vi "Disable All Buttons(Motor Movement).vi"(8 "error in (no error)":errorcluster, 11 "ZenGage v3.0 UI in":refnum<class "ZenGage v3.0 UI.lvclass">) -> (0 "error out":errorcluster, 3 "ZenGage v3.0 UI out":refnum<class "ZenGage v3.0 UI.lvclass">)   [LabVIEW 2015, in "ZenGage v3.0 UI.lvclass"]
uses:
  ZenGage v3.0 UI.lvclass
  ZenGage v3.0 UI.lvclass/ZenGage v3.0 UI.ctl
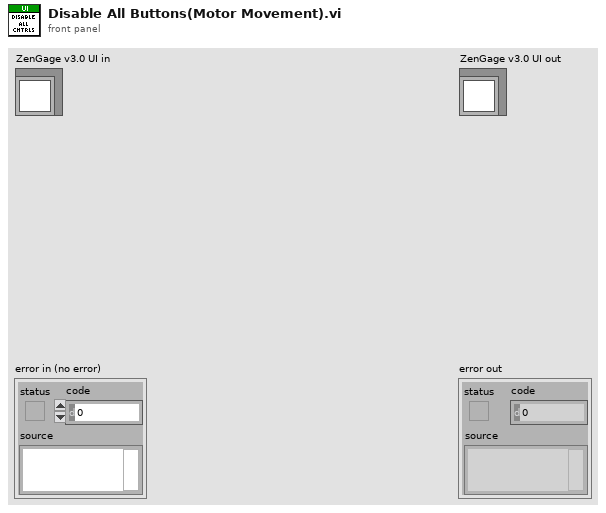
[diagram p1: front panel]
types:
  T1 = enum32{"Analytics", "Blank", "Diagnostics", "Run", "Edit Tolerance Settings"}
  T2 = enum8{"Enabled", "Disabled", "Disabled and Grayed Out"}
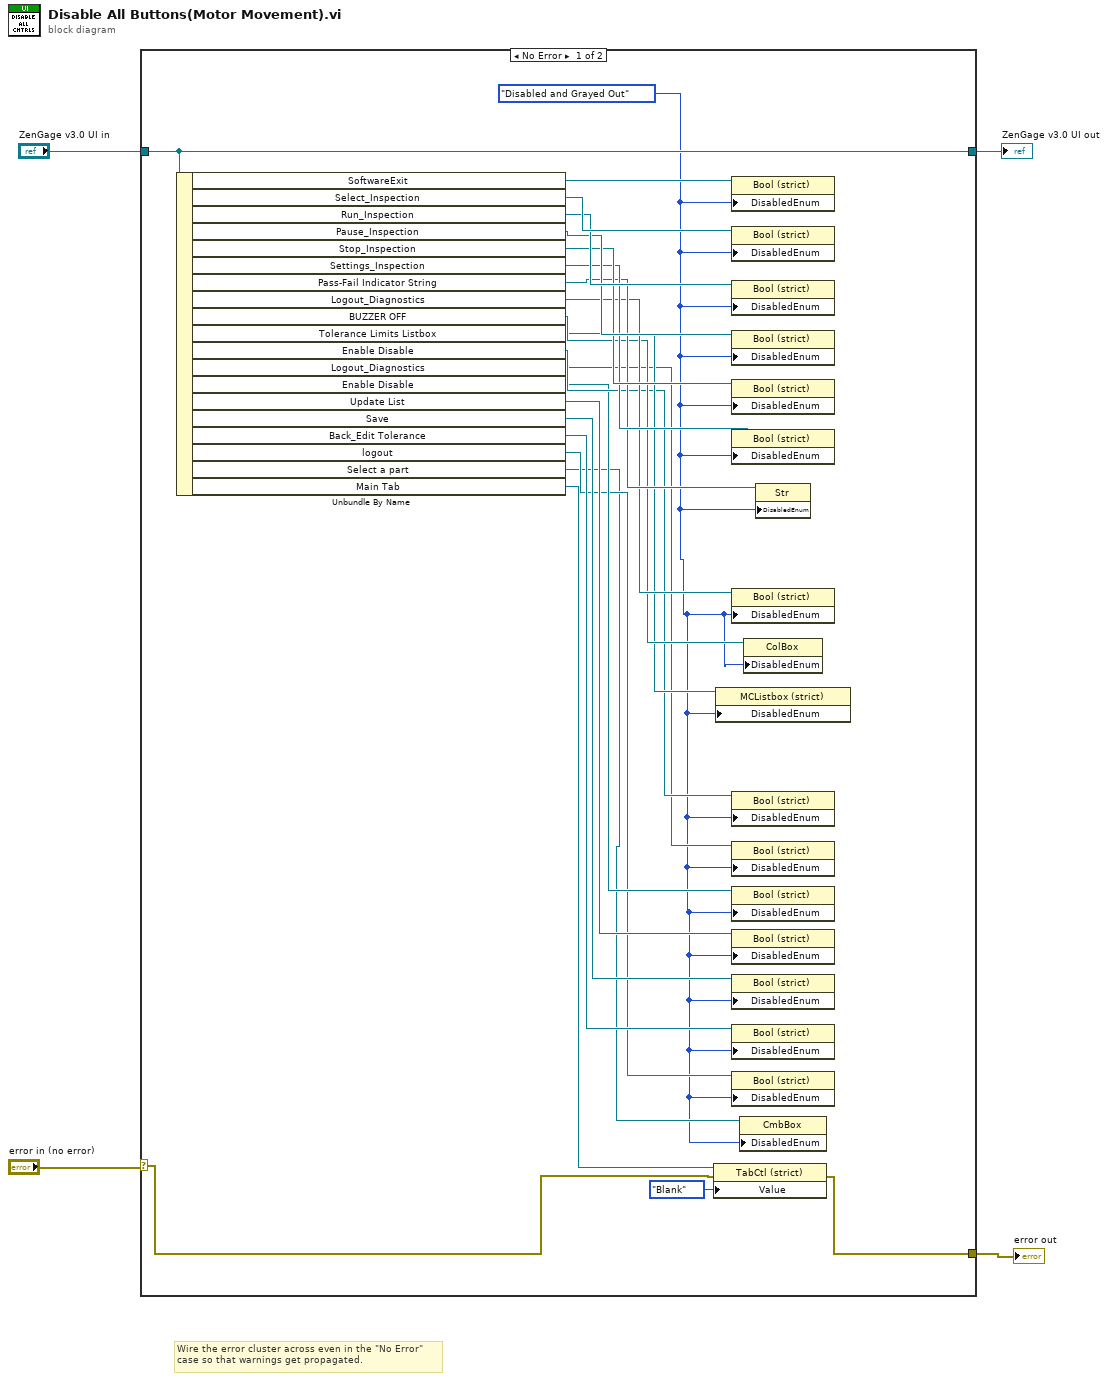
[diagram p0: block diagram]
diagram:
  # "Wire the error cluster across even in the \"No Error\"\ncase so that warnings get propagated."
  n1 = case shown="No Error" "error in (no error)" {
    selector: "error in (no error)" -> [w8 w30]
    tunnel: [w7 w30] -> w3
    tunnel: [w28 w29] -> w1
    tunnel: "ZenGage v3.0 UI in" -> [w28 w29]
    frame No Error {
      w5 = T2."Disabled and Grayed Out" ("Disabled")
      n2 = Unbundle By Name(w28) -> ("SoftwareExit"=w27:refnum<vi>, "Select_Inspection"=w26:refnum<vi>, "Run_Inspection"=w25:refnum<vi>, "Pause_Inspection"=w24:refnum<vi>, "Stop_Inspection"=w23:refnum<vi>, "Settings_Inspection"=w22:refnum<vi>, "Pass-Fail Indicator String"=w21:refnum<vi>, "Logout_Diagnostics"=w20:refnum<vi>, "BUZZER OFF"=w19:refnum<vi>, "Tolerance Limits Listbox"=w18:refnum<vi>, "Enable Disable"=w17:refnum<vi>, "Logout_Diagnostics"=w16:refnum<vi>, "Enable Disable"=w15:refnum<vi>, "Update List"=w14:refnum<vi>, "Save"=w13:refnum<vi>, "Back_Edit Tolerance"=w12:refnum<vi>, "logout"=w11:refnum<vi>, "Select a part"=w10:refnum<vi>, "Main Tab"=w9:refnum<vi>)
      n3 = property class="TabCtl (strict)"(reference=w9, error in=w8, "Value"=T1."Blank") -> (error out=w7:errorcluster)  [unwired: 1 out]
      n4 = property class="MCListbox (strict)"(reference=w18, "DisabledEnum"=w5) -> ()  [unwired: 1 in, 2 out]
      n5 = property class="Bool (strict)"(reference=w27, "DisabledEnum"=w5) -> ()  [unwired: 1 in, 2 out]
      n6 = property class="Bool (strict)"(reference=w26, "DisabledEnum"=w5) -> ()  [unwired: 1 in, 2 out]
      n7 = property class="Bool (strict)"(reference=w25, "DisabledEnum"=w5) -> ()  [unwired: 1 in, 2 out]
      n8 = property class="Bool (strict)"(reference=w24, "DisabledEnum"=w5) -> ()  [unwired: 1 in, 2 out]
      n9 = property class="Bool (strict)"(reference=w23, "DisabledEnum"=w5) -> ()  [unwired: 1 in, 2 out]
      n10 = property class="Bool (strict)"(reference=w22, "DisabledEnum"=w5) -> ()  [unwired: 1 in, 2 out]
      n11 = property class="Bool (strict)"(reference=w20, "DisabledEnum"=w5) -> ()  [unwired: 1 in, 2 out]
      n12 = property class="Bool (strict)"(reference=w17, "DisabledEnum"=w5) -> ()  [unwired: 1 in, 2 out]
      n13 = property class="Bool (strict)"(reference=w16, "DisabledEnum"=w5) -> ()  [unwired: 1 in, 2 out]
      n14 = property class="Bool (strict)"(reference=w15, "DisabledEnum"=w5) -> ()  [unwired: 1 in, 2 out]
      n15 = property class="Bool (strict)"(reference=w14, "DisabledEnum"=w5) -> ()  [unwired: 1 in, 2 out]
      n16 = property class="Bool (strict)"(reference=w13, "DisabledEnum"=w5) -> ()  [unwired: 1 in, 2 out]
      n17 = property class="Bool (strict)"(reference=w12, "DisabledEnum"=w5) -> ()  [unwired: 1 in, 2 out]
      n18 = property class="Bool (strict)"(reference=w11, "DisabledEnum"=w5) -> ()  [unwired: 1 in, 2 out]
      n19 = property class="CmbBox"(reference=w10, "DisabledEnum"=w5) -> ()  [unwired: 1 in, 2 out]
      n20 = property class="ColBox"(reference=w19, "DisabledEnum"=w5) -> ()  [unwired: 1 in, 2 out]
      n21 = property class="Str"(reference=w21, "DisabledEnum"=w5) -> ()  [unwired: 1 in, 2 out]
    }
    frame Error {
    }
  }
  "error out" <- w3
  "ZenGage v3.0 UI out" <- w1
